vi "merFISH_autofocus_signal_search_fine.vi"(5 "error in":errorcluster, 6 "QPD ref":T1, 7 "Slope":dbl, 8 "queue piezo":refnum<queue>) -> (0 "error out":errorcluster, 3 "Ref found?":bool)   [LabVIEW 2015]
uses:
  CONTROLS/Q_MCL_piezo_element.ctl
  <vilib>/Utility/miscctls.llb/LVCursorListTypeDef.ctl
  GLOBAL/Global_MCL_piezo.vi
  GLOBAL/Global_FPGA.vi
panel:
  out "XY Graph":cluster{"X":dbl, "Y":dbl}[](graph)
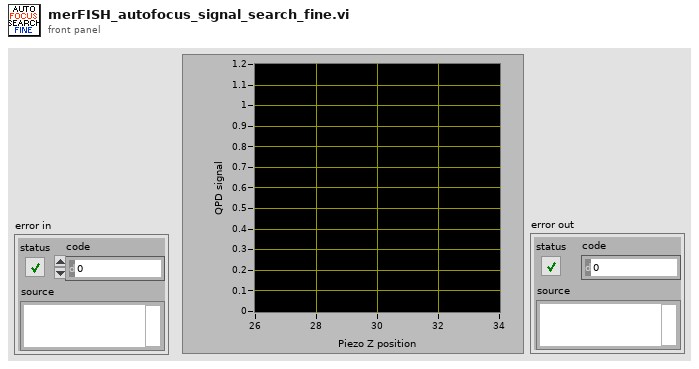
[diagram p1: front panel]
types:
  T1 = cluster{"X":sgl, "Y":sgl, "SUM":sgl, "count":u32}
  T2 = typedef "Q_MCL_piezo_element.ctl" = cluster{"variant":variant, "Instruction":enum16{"Piezo_idle", "Piezo_initialize", "Piezo_error", "Piezo_security_stop", "Piezo_read_z", "Piezo_move_z", "Piezo_keyboard_move", "Piezo_close_autofocus_calibration_ramp", "Piezo_change_init_state", "Piezo_init_autofocus", "Piezo_init_autofocus_merFISH_TL", "Piezo_autofocus", "Piezo_autofocus_merFISH_TL", "Piezo_stop_autofocus", "Piezo_stop_autofocus_merFISH_TL", "Piezo_autofocus_lost", "Piezo_resume_autofocus_merFISH_TL", "Piezo_check_z_position_merFISH_TL", "Piezo_init_ramp", "Piezo_move_z_ramp", "Piezo_close_ramp", "Piezo_close_merFISH", "Piezo_stop"}}
  T3 = typedef "LVCursorListTypeDef.ctl" = cluster{"Name":string, "Color":u32, "Style":u8, "Point Style":u8, "Name Visible":bool, "Allow Drag":bool, "Cursor Mode":u32, "Plot":i32, "Index":i32, "Position":cluster{"X":dbl, "Y":dbl}, "X Scale":u32, "Y Scale":u32, "Watch Plots":i32[], "Watch All Plots":bool, "Plot Area":i32, "Label Offset":cluster{"X":dbl, "Y":dbl}}[]
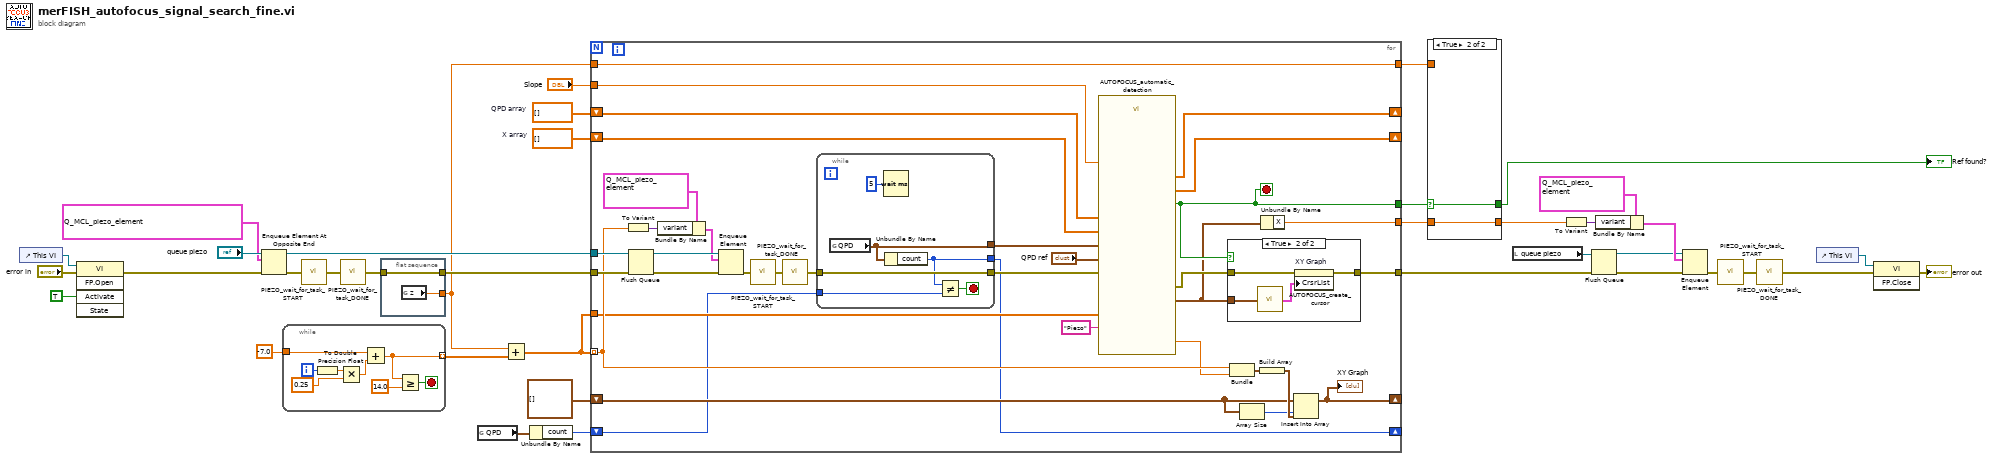
[diagram p0: block diagram]
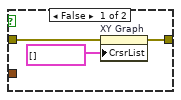
[diagram p3: hidden frame]
diagram:
  w13 = dbl[] []  # QPD array
  w11 = dbl[] []  # X array
  n1 = control-ref of="This VI"() -> (w20:refnum<vi>)
  n2 = invoke class="VI" method="FP.Open"(reference=w20, error in="error in", "Activate"=TRUE ("Activate?")) -> (error out=w17:errorcluster)  [unwired: 2 in, 4 out]
  n3 = Enqueue Element At Opposite End(queue="queue piezo", element=T2 {"variant"=variant, "Instruction"=enum."Piezo_check_z_position_merFISH_TL"}, error in (no error)=w17) -> (queue out=w33:refnum<queue>, error out=w37:errorcluster)  [unwired: 1 in, 1 out]
  n4 = while {
    tunnel: -7.0 -> [w43]
    tunnel: [w41] -> w34 mode=indexing
    i -> [w46]
    stop <- w39 stop-if-true
    n5 = To Double Precision Float(number=w46) -> (double precision float=w44:dbl)
    n6 = Multiply(x=w44, y=0.25) -> (x*y=w42:dbl)
    n7 = Add(x=w43, y=w42) -> (x+y=w41:dbl)
    n8 = Greater Or Equal?(x=w41, y=14.0) -> (x >= y?=w39:bool)
  }
  n9 = call "PIEZO_wait_for_task_START.vi"("error in"=w37) -> ("error out"=w36:errorcluster)
  n10 = call "PIEZO_wait_for_task_DONE.vi"("error in"=w36) -> ("error out"=w35:errorcluster)
  n11 = flat-sequence {
    tunnel: w35 -> [w48]
    tunnel: [w48] -> w32
    tunnel: [w47] -> w9
    frame #0 {
      n12 = global read "Global_MCL_piezo.vi" "z"() -> (w47:dbl)
    }
  }
  n13 = global read "Global_FPGA.vi" "QPD"() -> (w2:T1)
  n14 = Add(x=w9, y=w34) -> (x+y=w10:dbl[])
  n15 = Unbundle By Name(w2) -> ("count"=w1:u32)
  n16 = for {
    tunnel: w10 -> [w73] mode=indexing
    tunnel: w33 -> [w83]
    tunnel: w32 -> [w74]
    shift-right: [w76] -> _
    shift-left: cluster{dbl, "norm":dbl}[] [] ("appended array") -> [w77]
    tunnel: [w62] -> w26
    tunnel: "Slope" -> [w68]
    shift-right: [w65] -> _
    shift-left: w13 -> [w66]
    shift-right: [w64] -> _
    shift-left: w11 -> [w67]
    tunnel: [w61] -> w7
    tunnel: w10 -> [w59]
    tunnel: w9 -> [w58]
    tunnel: [w58] -> w8
    tunnel: [w56] -> w5
    shift-right: [w50] -> _
    shift-left: w1 -> [w52]
    stop <- w61 stop-if-true
    n17 = To Variant(anything=w73) -> (Variant=w80:variant)
    n18 = Flush Queue(queue=w83, error in (no error)=w74) -> (queue out=w82:refnum<queue>, error out=w81:errorcluster)  [unwired: 1 out]
    n19 = Bundle By Name(cluster=T2 {"variant"=variant, "Instruction"=enum."Piezo_move_z"} ("element"), "variant"=w80) -> (w72:T2)
    n20 = Enqueue Element(queue=w82, element=w72, error in (no error)=w81) -> (error out=w69:errorcluster)  [unwired: 1 in, 2 out]
    n21 = call "PIEZO_wait_for_task_START.vi"("error in"=w69) -> ("error out"=w70:errorcluster)
    n22 = call "PIEZO_wait_for_task_DONE.vi"("error in"=w70) -> ("error out"=w54:errorcluster)
    n23 = while {
      tunnel: w54 -> [w89]
      tunnel: [w89] -> w53
      tunnel: w52 -> [w87]
      tunnel: [w86] -> w51
      tunnel: [w84] -> w50
      stop <- w85 stop-if-true
      n24 = global read "Global_FPGA.vi" "QPD"() -> (w86:T1)
      n25 = Wait (ms)(milliseconds to wait=u32 5) -> ()  [unwired: 1 out]
      n26 = Unbundle By Name(w86) -> ("count"=w84:u32)
      n27 = Not Equal?(x=w84, y=w87) -> (x != y?=w85:bool)
    }
    n28 = call "AUTOFOCUS_automatic_detection.vi"("X array"=w67, "QPD array"=w66, "Stage type"="Piezo", "QPD ref"="QPD ref", "Slope"=w68, "QPD"=w51, "error in"=w53, "Search array"=w59) -> ("QPD array out"=w65:dbl[], "X array out"=w64:dbl[], "Cursor"=w57:cluster{"X":dbl, "Y":dbl}, "Setpoint detected"=w61:bool, "norm"=w60:dbl, "error out"=w63:errorcluster)  [unwired: 2 in]
    n29 = case shown="True" w61 {
      tunnel: w63 -> [w92 w95]
      tunnel: [w91 w93] -> w62
      tunnel: w57 -> [_ w96]
      frame False {
        n30 = property on="XY Graph" class="XYGraph (strict)"(error in=w92, "CrsrList"=T3 [] ("Cursor List")) -> (error out=w91:errorcluster)  [unwired: 1 in, 1 out]
      }
      frame True {
        n31 = call "AUTOFOCUS_create_cursor.vi"("Position"=w96) -> ("cursor array"=w94:T3)
        n32 = property on="XY Graph" class="XYGraph (strict)"(error in=w95, "CrsrList"=w94) -> (error out=w93:errorcluster)  [unwired: 1 in, 1 out]
      }
    }
    n33 = Bundle(w73, "norm"=w60) -> (w79:cluster{dbl, "norm":dbl})  [unwired: 1 in]
    n34 = Array Size(array=w77) -> (size(s)=w75:i32)
    n35 = Build Array(w79) -> (w78:cluster{dbl, "norm":dbl}[])
    n36 = Unbundle By Name(w57) -> ("X"=w56:dbl)
    n37 = Insert Into Array(array=w77, index=w75, new element=w78) -> (w76:cluster{dbl, "norm":dbl}[])
    "XY Graph" <- w76
  }
  n38 = case shown="True" w7 {
    selector: w7 -> [w98 w99]
    tunnel: w5 -> [_ w100]
    tunnel: [w97 w100] -> w4
    tunnel: w8 -> [w97 _]
    tunnel: [w98 w99] -> w6
    frame False {
    }
    frame True {
    }
  }
  "Ref found?" <- w6
  n39 = local read "queue piezo"() -> (w24:refnum<queue>)
  n40 = To Variant(anything=w4) -> (Variant=w30:variant)
  n41 = Flush Queue(queue=w24, error in (no error)=w26) -> (queue out=w27:refnum<queue>, error out=w28:errorcluster)  [unwired: 1 out]
  n42 = Bundle By Name(cluster=T2 {"variant"=variant, "Instruction"=enum."Piezo_move_z"} ("element"), "variant"=w30) -> (w29:T2)
  n43 = Enqueue Element(queue=w27, element=w29, error in (no error)=w28) -> (error out=w21:errorcluster)  [unwired: 1 in, 2 out]
  n44 = call "PIEZO_wait_for_task_START.vi"("error in"=w21) -> ("error out"=w22:errorcluster)
  n45 = call "PIEZO_wait_for_task_DONE.vi"("error in"=w22) -> ("error out"=w14:errorcluster)
  n46 = control-ref of="This VI"() -> (w16:refnum<vi>)
  n47 = invoke class="VI" method="FP.Close"(reference=w16, error in=w14) -> (error out=→"error out":errorcluster)  [unwired: 1 in, 2 out]
